vi "create.vi"(8 "error in (no error)":errorcluster, 10 "ref":u64) -> (0 "error out":errorcluster, 3 "Value out":refnum<class "Value.lvclass">)   [LabVIEW 2020, in "toml_edit.lvlib" / "Value.lvclass"]
uses:
  Value.lvclass
  Value.lvclass/Value.ctl
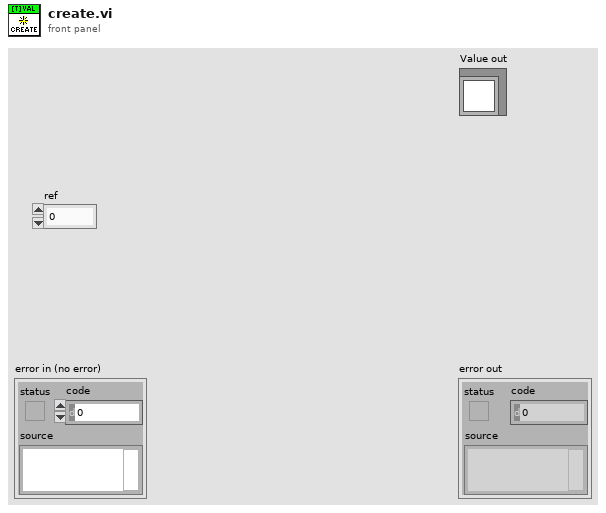
[diagram p1: front panel]
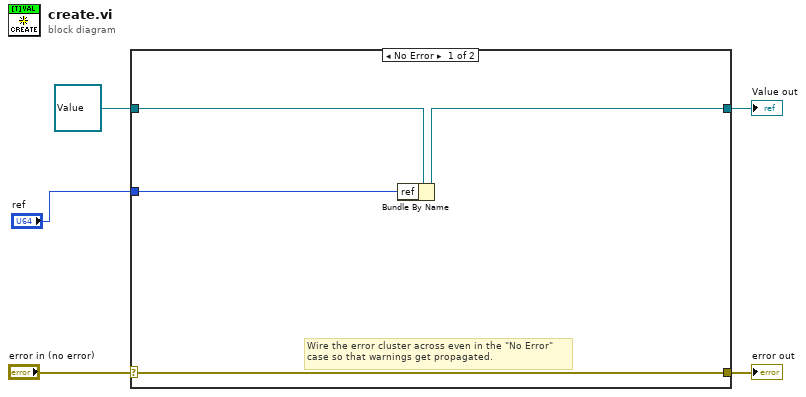
[diagram p0: block diagram]
diagram:
  n1 = case shown="No Error" "error in (no error)" {
    selector: "error in (no error)" -> [w8 w11]
    tunnel: [w8 w11] -> w4
    tunnel: [w7 w10] -> w2
    tunnel: refnum<class "Value.lvclass"> refnum ("Value in") -> [w9 w10]
    tunnel: "ref" -> [w6 _]
    frame No Error {
      # "Wire the error cluster across even in the \"No Error\"\ncase so that warnings get propagated."
      n2 = Bundle By Name(cluster=w9, "ref"=w6) -> (w7:refnum<class "Value.lvclass">)
    }
    frame Error {
    }
  }
  "error out" <- w4
  "Value out" <- w2
